vi "Dialog_Spectr2 (SubVI).vi"() -> ()   [LabVIEW 2017]
doc: "Use this template to build a user interface event handler design pattern. Use this pattern for dialog boxes and other user interfaces. You also can create and execute user-defined events that the VI can handle the same way as user interface events."
uses:
  <vilib>/Analysis/4window.llb/windowTd.ctl
  Global_SNK3_HF.vi
  <vilib>/measure/maspectr.llb/FFT Spectrum (Mag-Phase) for 1 Chan.vi
  <vilib>/measure/NI_MAPro.lvlib
  <vilib>/Analysis/NI_AALPro.lvlib
panel:
  in  "Номер такта":u8
  in  "timeout":i32=500 min=200 max=2000 step=1
  out "Спектр":cluster{"f0":dbl, "df":dbl, "magnitude":dbl[]}(graph)
  in  "averaging parameters":T1={"averaging mode"=enum."RMS averaging", "weighting mode"=enum."Exponential", "number of averages"=8} {"number of averages" min=1}
  in  "window":T2=6 items=["Rectangle"=0, "Hanning"=1, "Hamming"=2, "Blackman-Harris"=3, "Exact Blackman"=4, "Blackman"=5, "Flat Top"=6, "4 Term B-Harris "=7, "7 Term B-Harris"=8, "Low Sidelobe"=9, "Blackman Nuttall"=11, "Triangle"=30, "Bartlett-Hanning"=31, "Bohman"=32, "Parzen"=33, "Welch"=34, "Kaiser"=60, "Dolph-Chebyshev"=61, "Gaussian"=62]
  in  "stop":bool
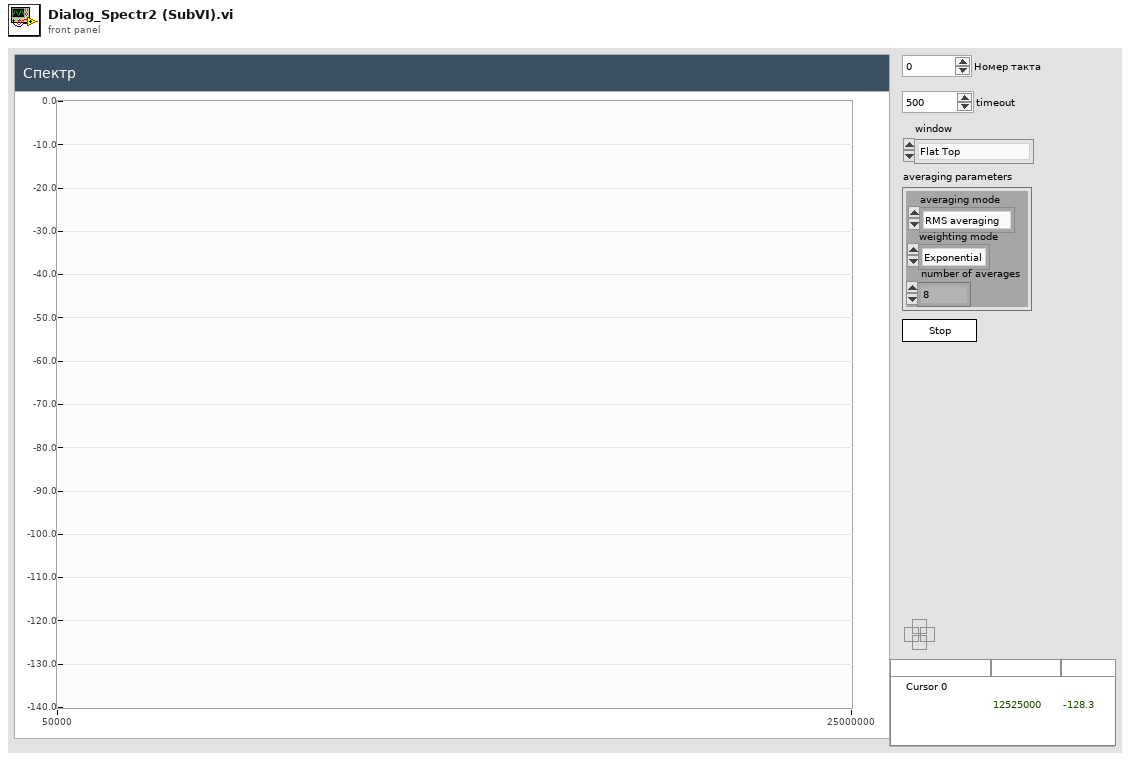
[diagram p1: front panel]
types:
  T1 = cluster{"averaging mode":enum16{"No averaging", "Vector averaging", "RMS averaging", "Peak hold"}, "weighting mode":enum16{"Linear", "Exponential"}, "number of averages":u32}
  T2 = typedef "NI_AALPro.lvlib/windowTd.ctl" = u32
  T3 = cluster{"dB On (F)":bool, "unwrap phase (F)":bool, "convert to degree (F)":bool}
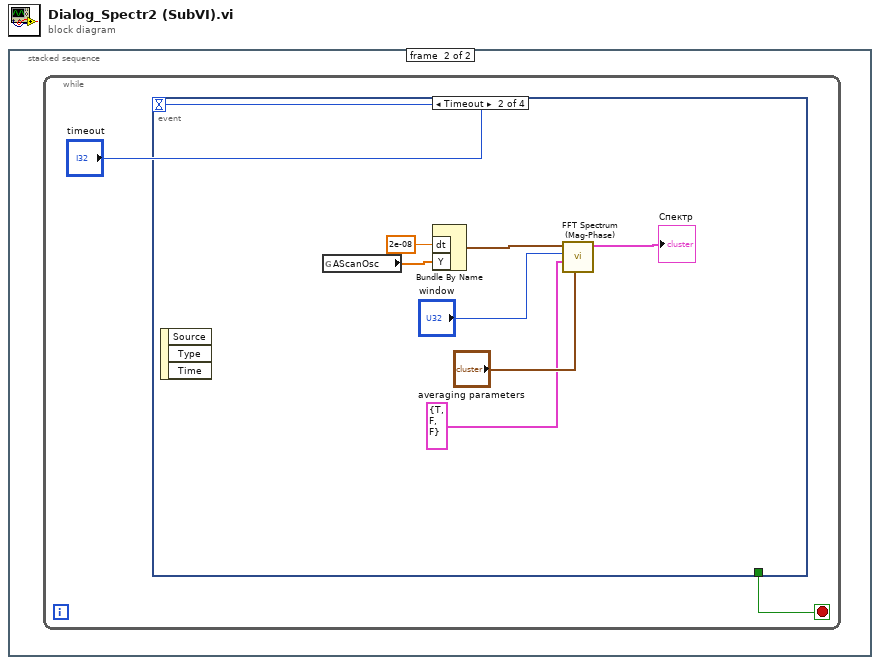
[diagram p0: block diagram]
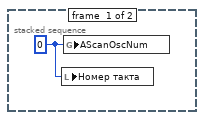
[diagram p2: hidden frame]
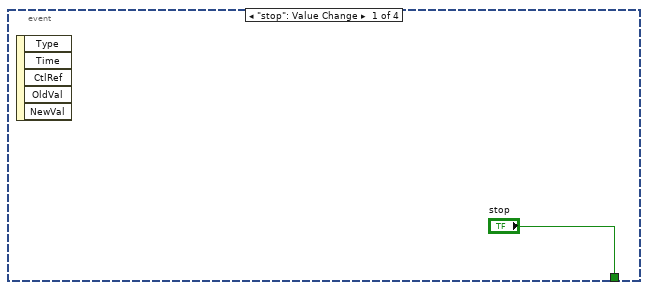
[diagram p3: hidden frame]
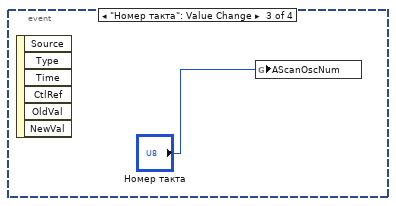
[diagram p4: hidden frame]
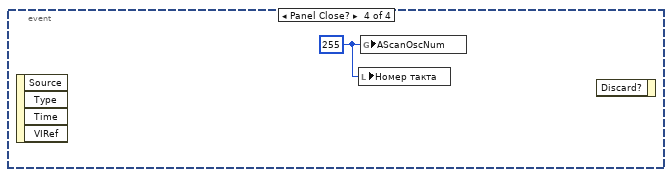
[diagram p5: hidden frame]
diagram:
  n1 = stacked-sequence {
    frame #0 {
      w1 = u8 0 ("AScanOscNum")
      n2 = local write "Номер такта"(w1) -> ()
      n3 = global write "Global_SNK3_HF.vi" "AScanOscNum"(w1) -> ()
    }
    frame #1 {
      n4 = while {
        stop <- w3 stop-if-true
        n5 = event shown="[1] Timeout" {
          selector: _ -> [_ _ _ _]
          dyn-events: _ -> [_ _ _ _]
          timeout: "timeout" -> [_ _ _ _]
          tunnel: ["stop" _ _ _] -> w3
          event "stop": Value Change {
            n6 = event-data() -> ()  [unwired: 1 in, 5 out]
          }
          event Timeout {
            n7 = event-data() -> ()  [unwired: 1 in, 3 out]
            n8 = global read "Global_SNK3_HF.vi" "AScanOsc"() -> (w11:dbl[])
            n9 = Bundle By Name("dt"=2e-08, "Y"=w11) -> (w10:waveform(dbl))  [unwired: 1 in]
            n10 = call-poly <vilib>:"FFT Spectrum (Mag-Phase).vi"("averaging parameters"="averaging parameters", "view"=T3 {"dB On (F)"=TRUE, "unwrap phase (F)"=FALSE, "convert to degree (F)"=FALSE}, "window"="window", "time signal"=w10) -> ("magnitude"=→"Спектр":cluster{"f0":dbl, "df":dbl, "magnitude":dbl[]})  [unwired: 3 in, 4 out]
          }
          event "Номер такта": Value Change {
            n11 = event-data() -> ()  [unwired: 1 in, 6 out]
            n12 = global write "Global_SNK3_HF.vi" "AScanOscNum"("Номер такта") -> ()
          }
          event Panel Close? {
            w13 = u8 255 ("AScanOscNum")
            n13 = event-data() -> ()  [unwired: 1 in, 4 out]
            n14 = local write "Номер такта"(w13) -> ()
            n15 = global write "Global_SNK3_HF.vi" "AScanOscNum"(w13) -> ()
            n16 = event-data() -> ()  [unwired: 2 in, 1 out]
          }
        }
      }
    }
  }
